vi "GetActiveScheduleName.vi"(11 "Target Ref":T1 format="%.0x") -> (3 "Value":string)   [LabVIEW 2016, in "LIN Frame Protection Addon System Explorer.lvlib"]
uses:
  LIN Frame Protection Addon System Explorer.lvlib
  <vilib>/NI Veristand/Custom Device API/Custom Device Item Ref.ctl
  <vilib>/NI Veristand/Custom Device API/Get Item Property (String).vi
  <vilib>/NI Veristand/Custom Device API/Custom Device API.lvlib
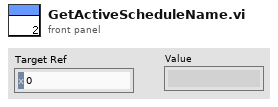
[diagram p1: front panel]
types:
  T1 = typedef "Custom Device API.lvlib/Custom Device Item Ref.ctl" = u64
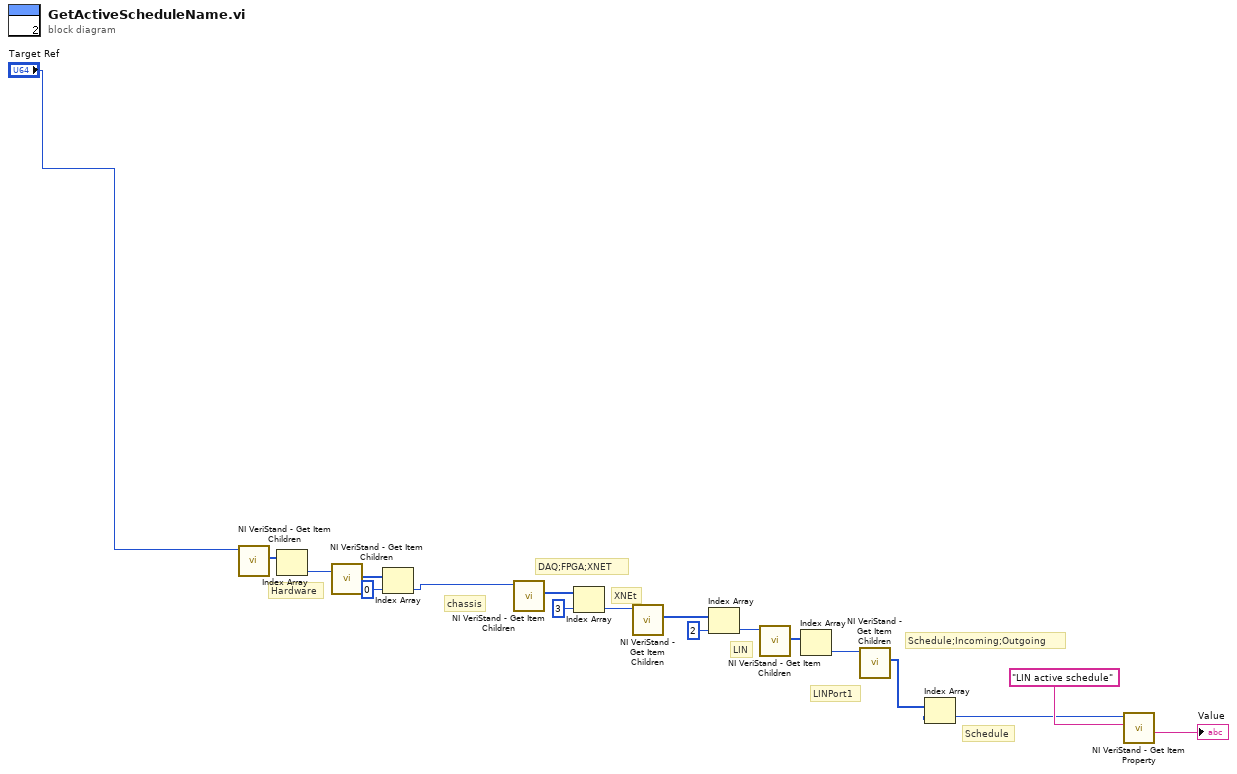
[diagram p0: block diagram]
diagram:
  # "Schedule"
  # "Schedule;Incoming;Outgoing"
  # "LINPort1"
  # "LIN"
  # "DAQ;FPGA;XNET"
  # "XNEt"
  # "chassis"
  # "Hardware"
  n1 = call <vilib>:"NI VeriStand - Get Item Children.vi"("Item Ref in"="Target Ref") -> ("Child Refs"=w17:T1[])  [unwired: 7 in, 3 out]
  n2 = Index Array(array=w17) -> (element=w16:T1)  [unwired: 1 in]
  n3 = call <vilib>:"NI VeriStand - Get Item Children.vi"("Item Ref in"=w16) -> ("Child Refs"=w15:T1[])  [unwired: 7 in, 3 out]
  n4 = Index Array(array=w15, index=0) -> (element=w13:T1)
  n5 = call <vilib>:"NI VeriStand - Get Item Children.vi"("Item Ref in"=w13) -> ("Child Refs"=w10:T1[])  [unwired: 7 in, 3 out]
  n6 = Index Array(array=w10, index=3) -> (element=w11:T1)
  n7 = call <vilib>:"NI VeriStand - Get Item Children.vi"("Item Ref in"=w11) -> ("Child Refs"=w9:T1[])  [unwired: 7 in, 3 out]
  n8 = Index Array(array=w9, index=2) -> (element=w7:T1)
  n9 = call <vilib>:"NI VeriStand - Get Item Children.vi"("Item Ref in"=w7) -> ("Child Refs"=w6:T1[])  [unwired: 7 in, 3 out]
  n10 = Index Array(array=w6) -> (element=w5:T1)  [unwired: 1 in]
  n11 = call <vilib>:"NI VeriStand - Get Item Children.vi"("Item Ref in"=w5) -> ("Child Refs"=w4:T1[])  [unwired: 7 in, 3 out]
  n12 = Index Array(array=w4) -> (element=w1:T1)  [unwired: 1 in]
  n13 = call-poly <vilib>:"NI VeriStand - Get Item Property.vi"("Property Name"="LIN active schedule", "Item Ref in"=w1) -> ("Value"=→"Value":string)  [unwired: 6 in, 3 out]
